vi "CaseStructure - Add Frame.vi"(8 "error in (no error)":errorcluster, 9 "Case Name":string, 10 "Reference Frame Index":i32, 11 "CaseStructure in":refnum<vi>) -> (0 "error out":errorcluster, 2 "Add Frame":refnum<vi>, 3 "CaseStructure out":refnum<vi>)   [LabVIEW 2017, in "csmHelper-CaseStructure.lvlib"]
doc: "-- <b>Controls</b> --\n- <b>Case Name</b>:\n- <b>Reference Frame Index</b>:\n- <b>CaseStructure in</b>:\n\n-- <b>Indicators</b> --\n- <b>Add Frame</b>:\n- <b>CaseStructure out</b>:"
uses:
  csmHelper-CaseStructure.lvlib
  Communicable State Machine.lvlib
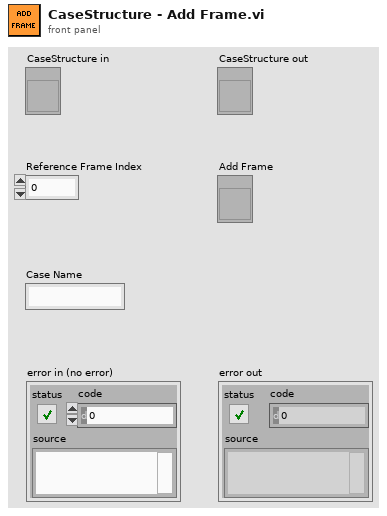
[diagram p1: front panel]
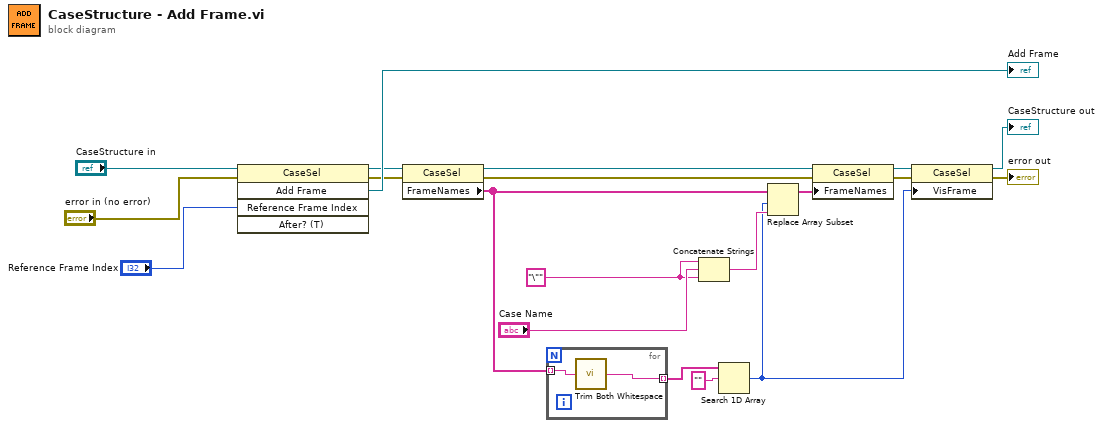
[diagram p0: block diagram]
diagram:
  w13 = "\"" ("string")
  n1 = invoke class="CaseSel" method="Add Frame"(reference="CaseStructure in", error in="error in (no error)", "Reference Frame Index"="Reference Frame Index") -> (reference out=w7:refnum<vi>, error out=w17:errorcluster, "Add Frame"=→"Add Frame":refnum<vi>)  [unwired: 2 in, 2 out]
  n2 = property class="CaseSel"(reference=w7, error in=w17) -> (reference out=w4:refnum<vi>, error out=w3:errorcluster, "FrameNames"=w6:string[])
  n3 = for {
    tunnel: [w22] -> w8 mode=indexing
    tunnel: w6 -> [w21] mode=indexing
    n4 = call "Trim Both Whitespace.vi"("string"=w21) -> ("trimmed string"=w22:string)  [unwired: 1 in]
  }
  n5 = Concatenate Strings(w13, "Case Name", w13) -> (w12:string)
  n6 = Search 1D Array(1D array=w8, element="") -> (index of element=w11:i32)  [unwired: 1 in]
  n7 = Replace Array Subset(array=w6, new element=w12, index=w11) -> (w5:string[])
  n8 = property class="CaseSel"(reference=w4, error in=w3, "FrameNames"=w5) -> (reference out=w10:refnum<vi>, error out=w9:errorcluster)
  n9 = property class="CaseSel"(reference=w10, error in=w9, "VisFrame"=w11) -> (reference out=→"CaseStructure out":refnum<vi>, error out=→"error out":errorcluster)
